vi "Resolve with Result.vi"(8 "error in (no error)":errorcluster, 10 "Result":variant, 11 "Promise in":refnum<class "Promise.lvclass">) -> (0 "error out":errorcluster)   [LabVIEW 2017, in "Futures.lvlib" / "Promise.lvclass"]
doc: "Resolves the promise with a result.\n\nThe promise should be treated as invalid after this point and may throw errors if attempt to use it again."
uses:
  Promise.lvclass
  Promise.lvclass/Promise.ctl
  Task/Task.lvclass
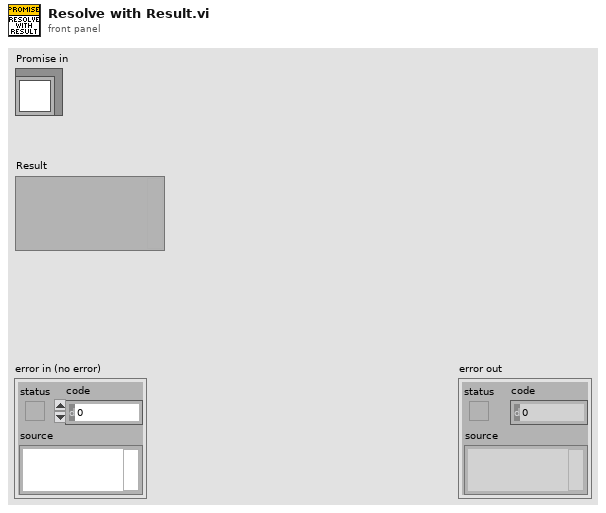
[diagram p1: front panel]
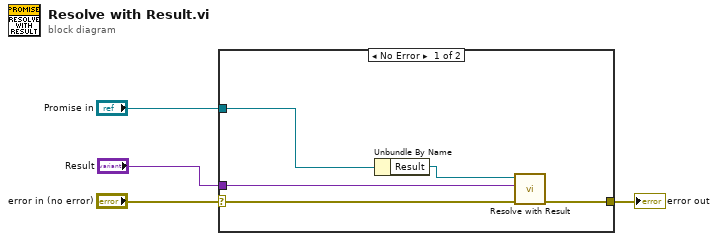
[diagram p0: block diagram]
diagram:
  n1 = case shown="No Error" "error in (no error)" {
    selector: "error in (no error)" -> [w9 w10]
    tunnel: [w8 w10] -> w3
    tunnel: "Promise in" -> [w7 _]
    tunnel: "Result" -> [w5 _]
    frame No Error {
      n2 = Unbundle By Name(w7) -> ("Result"=w6:refnum<class "Task.lvclass">)
      n3 = call "Resolve with Result.vi"("error in (no error)"=w9, "Result"=w5, "Result in"=w6) -> ("error out"=w8:errorcluster)  [unwired: 8 in]
    }
    frame Error {
    }
  }
  "error out" <- w3
